vi "Publisher Do.vi"(8 "error in (no error)":errorcluster, 10 "Publisher in":refnum<class "Publisher.lvclass">, 11 "Subscribe Msg":refnum<class "Targetted Msg.lvclass">) -> (0 "error out":errorcluster, 2 "Publisher out":refnum<class "Publisher.lvclass">)   [LabVIEW 2020, in "Publisher.lvlib" / "Targetted Msg.lvclass"]
doc: "This VI delivers the message to the actor by calling the appropriate method(s) on the actor.\n\nThe message is dropped if the forwarding failed."
uses:
  Targetted Msg.lvclass
  C:/Current projects/WS/Framework/Framework/Actors/Publisher/Publisher Messages/Sender Msg/Sender Msg.lvclass
  C:/Current projects/WS/Framework/Framework/Actors/Publisher/Publisher Messages/Publisher Msg/Publisher Msg.lvclass
  Publisher/Publisher.lvclass
  Sender Msg/Sender Msg.lvclass/Sender Msg.ctl
  Publisher Msg/Publisher Msg.lvclass/Publisher Msg.ctl
  Targetted Msg.lvclass/Targetted Msg.ctl
  PPL/HDH.Actor Framework.Core.Actor.lvlibp/1abvi3w/vi.lib/ActorFramework/Message/Message.lvclass
  Publisher Msg/Publisher Msg.lvclass
  Sender Msg/Sender Msg.lvclass
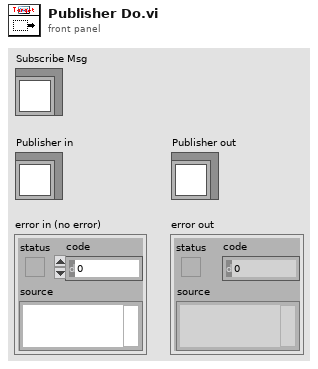
[diagram p1: front panel]
types:
  T1 = typedef "HDH.Actor Framework.Core.Actor.lvlibp/Message Enqueuer.lvclass/Message Priority.ctl" = enum16{"Low", "Normal", "High"}
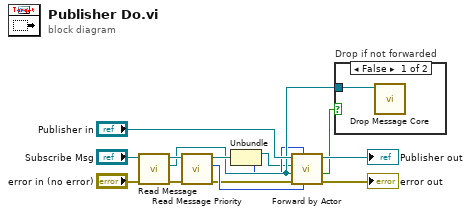
[diagram p0: block diagram]
diagram:
  n1 = call "Read Message.vi"("error in (no error)"="error in (no error)", "Sender Msg in"="Subscribe Msg") -> ("error out"=w6:errorcluster, "Message"=w3:refnum<class "Message.lvclass">, "Sender Msg out"=w4:refnum<class "Targetted Msg.lvclass">)  [unwired: 7 in]
  n2 = call "Read Message Priority.vi"("error in (no error)"=w6, "Publisher Msg in"=w4) -> ("error out"=w9:errorcluster, "Message Priority"=w12:T1, "Publisher Msg out"=w13:refnum<class "Targetted Msg.lvclass">)  [unwired: 7 in]
  n3 = Unbundle(w13) -> (w1:refnum<class "Actor.lvclass">, w2:i32)
  n4 = call "Forward by Actor.vi"("Message Priority (Normal)"=w12, "Target Actor index(-1, all)"=w2, "error in (no error)"=w9, "Message"=w3, "Target Actor"=w1, "Publisher in"="Publisher in") -> ("error out"=→"error out":errorcluster, "Message forwarded?"=w7:bool, "Publisher out"=→"Publisher out":refnum<class "Publisher.lvclass">)  [unwired: 3 in]
  n5 = case "Drop if not forwarded" shown="False" w7 {
    tunnel: w3 -> [w15 _]
    frame False {
      n6 = call-dynamic "Drop Message Core.vi"("Message in"=w15) -> ()  [unwired: 11 in]
    }
    frame True {
    }
  }
